vi "ModemTest.vi"() -> ()   [LabVIEW 2010]
uses:
  <vilib>/Instr/_visa.llb/VISA Configure Serial Port (Instr).vi
panel:
  in  "millisecond multiple":u32=1000
  out "write buffer":string="AQ3456789012345678901234"
  in  "stop":bool
  out "error out":errorcluster
  out "read buffer":string
  in  "*Com Port":refnum<visa-resource-name> caption="Com Port"
  in  "*Baud Rate":string(combo)="1200" caption="Baud Rate"
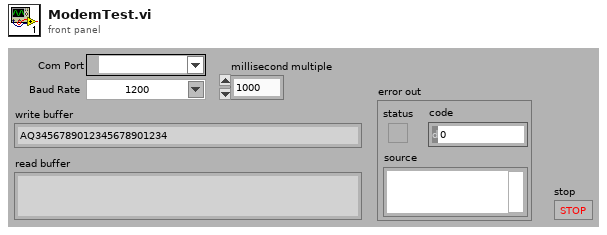
[diagram p1: front panel]
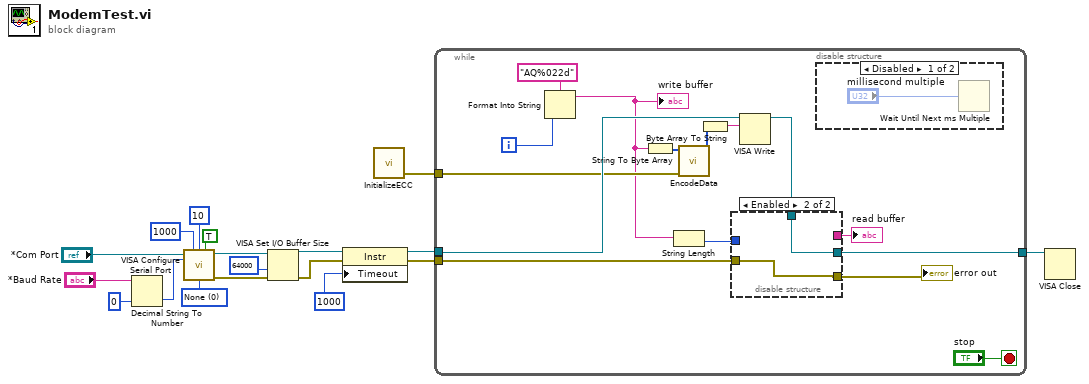
[diagram p0: block diagram]
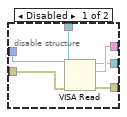
[diagram p3: hidden frame]
diagram:
  w16 = u16 0 items=["None", "XON/XOFF", "RTS/CTS", "XON/XOFF & RTS/CTS", "DTR/DSR", "XON/XOFF & DTR/DSR"] ("flow control (0:none)")
  n1 = Decimal String To Number(string="*Baud Rate", default (0L)=u32 0 ("default (0 I32)")) -> (number=w2:u32)  [unwired: 1 in, 1 out]
  n2 = call-poly "VISA Configure Serial Port"("VISA resource name"="*Com Port", "timeout (10sec)"=u32 1000, "termination char\n(0xA = '\\n' = LF)"=u8 10 ("termination char\n(0xA = '\\n' = LF)"), "Enable Termination\nChar (T)"=TRUE ("Enable Termination\nChar (T)"), "baud rate (9600)"=w2, "flow control (0:none)"=w16) -> ("VISA resource name out"=w7:refnum<visa-resource-name>, "error out"=w6:errorcluster)  [unwired: 3 in, 5 out]
  n3 = VISA Set I/O Buffer Size(VISA resource name=w7, size (4096)=u32 64000, error in (no error)=w6) -> (VISA resource name out=w14:refnum<visa-resource-name>, error out=w15:errorcluster)  [unwired: 1 out]
  n4 = property class="Instr"(reference=w14, error in=w15, "Timeout"=u32 1000 ("General Settings:Timeout Value")) -> (reference out=w5:refnum<visa-resource-name>, error out=w4:errorcluster)
  n5 = call "InitializeECC.vi"() -> ("Error Out"=w1:errorcluster)  [unwired: 11 in]
  n6 = while {
    tunnel: w5 -> [w27]
    tunnel: w4 -> [w28]
    tunnel: [w31] -> w3
    tunnel: w1 -> [w25]
    i -> [w21]
    stop <- "stop" stop-if-true
    n7 = Format Into String(format string="AQ%022d", w21) -> (resulting string=w19:string)  [unwired: 2 in, 1 out]
    "write buffer" <- w19
    n8 = String To Byte Array(string=w19) -> (unsigned byte array=w24:u8[])
    n9 = String Length(string=w19) -> (length=w29:i32)
    n10 = call "EncodeData.vi"("Error In"=w25, "Data In"=w24) -> ("Encoded Data Out"=w22:u8[])  [unwired: 8 in, 1 out]
    n11 = Byte Array To String(unsigned byte array=w22) -> (string=w23:string)
    n12 = VISA Write(VISA resource name=w27, write buffer=w23) -> (VISA resource name out=w26:refnum<visa-resource-name>)  [unwired: 1 in, 2 out]
    n13 = disable-structure shown="Enabled" {
      disable-tunnel: [w40 _] -> w33
      disable-tunnel: [w39 w41] -> w32
      disable-tunnel: [w38 w42] -> w31
      disable-tunnel: w29 -> [w37 _]
      disable-tunnel: w28 -> [w36 w41]
      disable-tunnel: w26 -> [w35 w42]
      frame Disabled {
        n14 = VISA Read(VISA resource name=w35, byte count=w37, error in (no error)=w36) -> (VISA resource name out=w38:refnum<visa-resource-name>, read buffer=w40:string, error out=w39:errorcluster)  [unwired: 1 out]
      }
      frame Enabled {
      }
    }
    "read buffer" <- w33
    "error out" <- w32
    n15 = disable-structure shown="Disabled" {
      frame Disabled {
        n16 = Wait Until Next ms Multiple(millisecond multiple="millisecond multiple") -> ()  [unwired: 1 out]
      }
      frame Enabled {
      }
    }
  }
  n17 = VISA Close(VISA resource name=w3) -> ()  [unwired: 1 in, 1 out]
